vi "Verify Power Down.vi"(0 "Measurement Configuration":T3={"Quick Power Down"=FALSE, "Pin Name"=[], "Source Mode"=[], "Start Value"=[], "Target Value"=[], "Compliance Limit"=[], "Sense Mode"=[], "Default Ramp Rate"=[], "Ramp Rate"=[], "Start Delay"=[], "Relative To"=[], "Transient Response"=[], "Data Capture"=FALSE, "Power line frequency"=1} {"Relative To" items=["Power sequence start", "Previous source start", "Previous source end"]; "Power line frequency" items=["50 Hz", "60 Hz"]; "Start Value" format="%#_6p"; "Transient Response" items=["Slow", "Normal", "Fast"]; "Sense Mode" items=["Local Sense", "Remote Sense"]; "Target Value" format="%#_6p"; "Source Mode" items=["DC Voltage", "DC Current"]; "Start Delay" format="%#_6p"; "Compliance Limit" format="%#_6p"; "Ramp Rate" format="%#_6p"}, 5 "Measurements":T1, 7 "PowerUP?":bool, 11 "error in (no error)":errorcluster) -> (4 "Error[]":string[](array[string]), 15 "error out":errorcluster)   [LabVIEW 2024, in "devicePowerSequencerCoreLogic.lvlib"]
doc: "Checks status of pins to verify the power up"
uses:
  devicePowerSequencerCoreLogic.lvlib
  Measurement Configuration.ctl
  controls/Source Mode.ctl
  controls/Sense Mode.ctl
  controls/Relative To.ctl
  controls/Transient Response.ctl
  controls/Power line frequency.ctl
  controls/Measurements.ctl
  controls/Voltage and Current Measurements.ctl
  <vilib>/Utility/error.llb/Clear Errors.vi
  Form Error Message.vi/4da3fa3f-d6a2-4c6b-9c9c-fc44bca91f7b.vi
  <vilib>/Utility/error.llb/Error Cluster From Error Code.vi
  Device Power Sequencer.lvlib
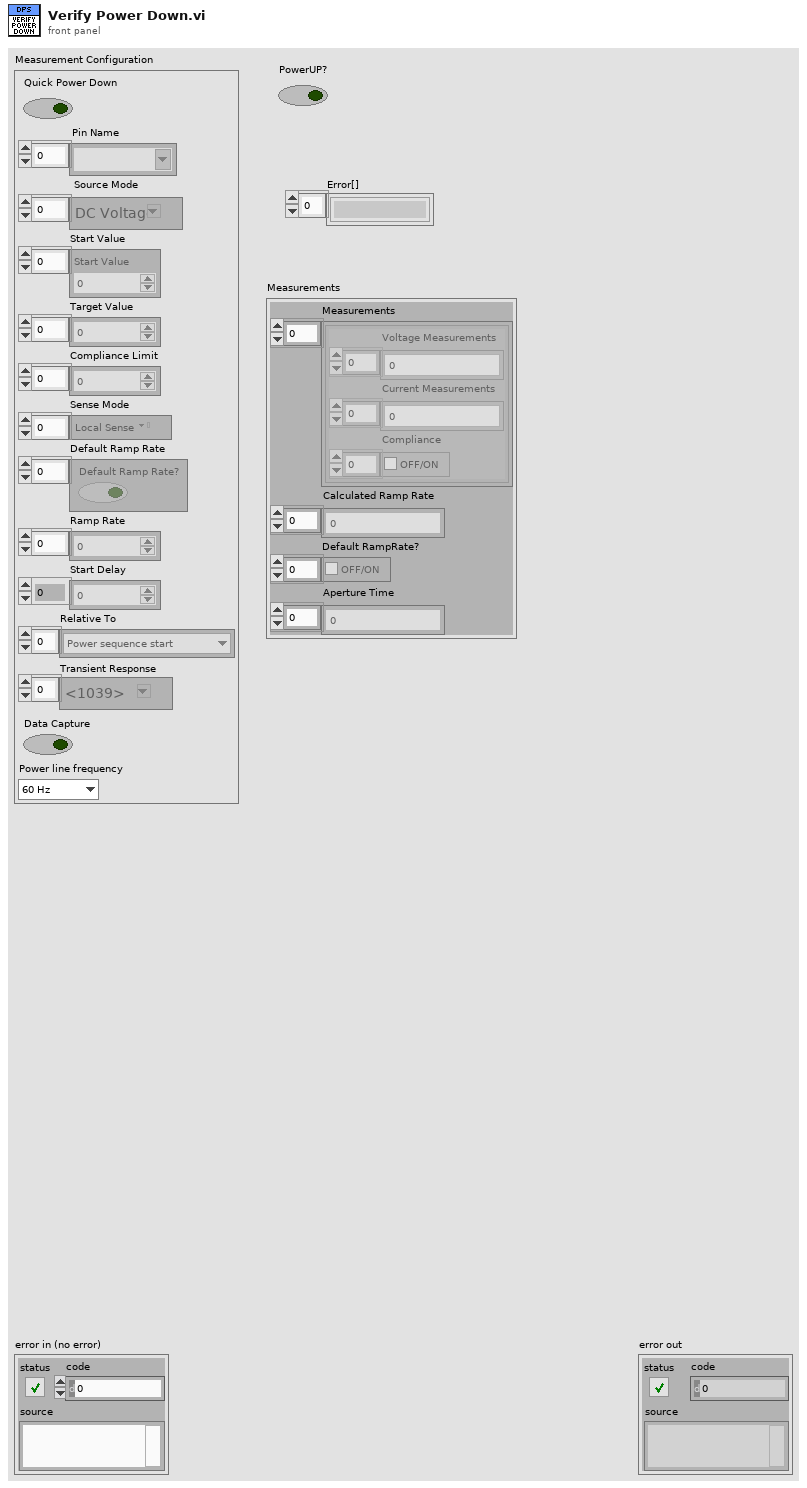
[diagram p1: front panel]
types:
  T1 = typedef "devicePowerSequencerCoreLogic.lvlib/Measurements.ctl" = cluster{"Measurements":T2[], "Calculated Ramp Rate":dbl[], "Default RampRate?":bool[], "Aperture Time":dbl[]}
  T2 = typedef "devicePowerSequencerCoreLogic.lvlib/Voltage and Current Measurements.ctl" = cluster{"Voltage Measurements":dbl[], "Current Measurements":dbl[], "Compliance":bool[]}
  T3 = typedef "Device Power Sequencer.lvlib/Measurement Configuration.ctl" = cluster{"Quick Power Down":bool, "Pin Name":string[], "Source Mode":T4[], "Start Value":dbl[], "Target Value":dbl[], "Compliance Limit":dbl[], "Sense Mode":T5[], "Default Ramp Rate":bool[], "Ramp Rate":dbl[], "Start Delay":dbl[], "Relative To":T6[], "Transient Response":T7[], "Data Capture":bool, "Power line frequency":T8}
  T4 = typedef "Device Power Sequencer.lvlib/Source Mode.ctl" = i32
  T5 = typedef "Device Power Sequencer.lvlib/Sense Mode.ctl" = i32
  T6 = typedef "Device Power Sequencer.lvlib/Relative To.ctl" = u32
  T7 = typedef "Device Power Sequencer.lvlib/Transient Response.ctl" = i32
  T8 = typedef "Device Power Sequencer.lvlib/Power line frequency.ctl" = u32
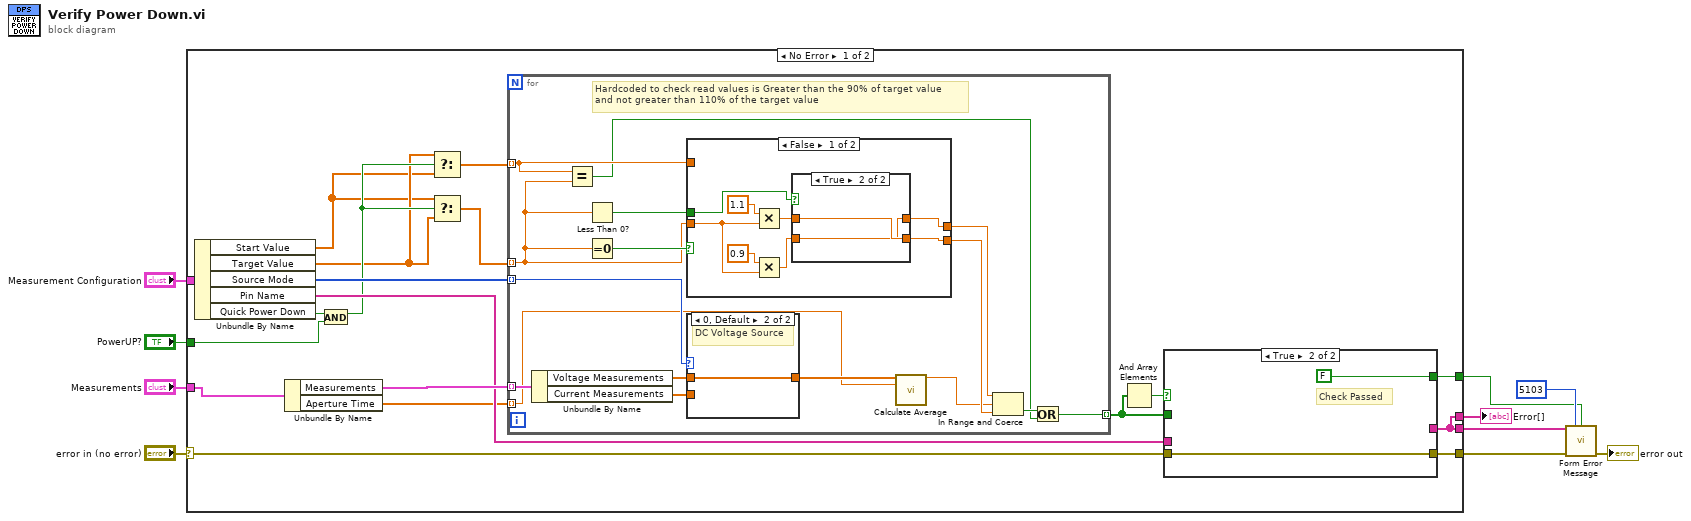
[diagram p0: block diagram]
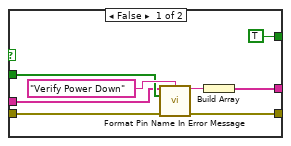
[diagram p2: hidden frame]
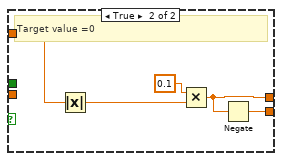
[diagram p4: hidden frame]
diagram:
  n1 = case shown="No Error" "error in (no error)" {
    selector: "error in (no error)" -> [w25 w75]
    tunnel: [w24 w75] -> w6
    tunnel: "Measurement Configuration" -> [w29 _]
    tunnel: "Measurements" -> [w27 _]
    tunnel: [w19 _] -> w4
    tunnel: [w20 _] -> w3
    tunnel: [w19 _] -> w2
    tunnel: "PowerUP?" -> [w14 _]
    frame No Error {
      n2 = Unbundle By Name(w29) -> ("Start Value"=w12:dbl[], "Target Value"=w13:dbl[], "Source Mode"=w28:T4[], "Pin Name"=w21:string[], "Quick Power Down"=w15:bool)
      n3 = Unbundle By Name(w27) -> ("Measurements"=w26:T2[], "Aperture Time"=w11:dbl[])
      n4 = And(x=w15, y=w14) -> (x .and. y?=w16:bool)
      n5 = Select(t=w13, s=w16, f=w12) -> (s? t:f=w18:dbl[])
      n6 = Select(t=w12, s=w16, f=w13) -> (s? t:f=w17:dbl[])
      n7 = for {
        tunnel: w26 -> [w55] mode=indexing
        tunnel: w28 -> [w54] mode=indexing
        tunnel: w17 -> [w44] mode=indexing
        tunnel: w18 -> [w45] mode=indexing
        tunnel: [w46] -> w22 mode=indexing
        tunnel: w11 -> [w41] mode=indexing
        # "Hardcoded to check read values is Greater than the 90% of target value\nand not greater than 110% of the target value"
        n8 = Unbundle By Name(w55) -> ("Voltage Measurements"=w52:dbl[], "Current Measurements"=w53:dbl[])
        n9 = Equal?(x=w45, y=w44) -> (x = y?=w43:bool)
        n10 = Less Than 0?(x=w44) -> (x < 0?=w48:bool)
        n11 = Equal To 0?(x=w44) -> (x = 0?=w49:bool)
        n12 = case shown="False" w49 {
          tunnel: [w59 w71] -> w51
          tunnel: [w58 w70] -> w50
          tunnel: w44 -> [w57 _]
          tunnel: w45 -> [_ w69]
          tunnel: w48 -> [w56 _]
          frame False {
            n13 = Multiply(x=1.1, y=w57) -> (x*y=w61:dbl)
            n14 = Multiply(x=0.9, y=w57) -> (x*y=w60:dbl)
            n15 = case shown="True" w56 {
              tunnel: w61 -> [w65 w67]
              tunnel: [w65 w66] -> w59
              tunnel: w60 -> [w64 w66]
              tunnel: [w64 w67] -> w58
              frame False {
              }
              frame True {
              }
            }
          }
          frame True {
            # "Target value =0"
            n16 = Absolute Value(x=w69) -> (abs(x)=w68:dbl)
            n17 = Multiply(x=0.1, y=w68) -> (x*y=w71:dbl)
            n18 = Negate(x=w71) -> (-x=w70:dbl)
          }
        }
        n19 = case shown="0, Default" w54 {
          tunnel: w53 -> [w73 _]
          tunnel: w52 -> [_ w74]
          tunnel: [w73 w74] -> w42
          frame 1 {
            # "DC Current Source"
          }
          frame 0, Default {
            # "DC Voltage Source"
          }
        }
        n20 = call "Calculate Average.vi"("Measurements"=w42, "Aperture Time"=w41) -> ("Average level"=w40:dbl)  [unwired: 13 in]
        n21 = In Range and Coerce(upper limit=w51, x=w40, lower limit=w50) -> (In Range?=w47:bool)  [unwired: 1 out]
        n22 = Or(x=w47, y=w43) -> (x .or. y?=w46:bool)
      }
      n23 = And Array Elements(Boolean array=w22) -> (logical AND=w23:bool)
      n24 = case shown="True" w23 {
        tunnel: [w36 w38] -> w24
        tunnel: [w35 _] -> w19
        tunnel: [TRUE ("Boolean") FALSE ("Boolean")] -> w20
        tunnel: w25 -> [w32 w38]
        tunnel: w22 -> [w31 _]
        tunnel: w21 -> [w30 _]
        frame False {
          n25 = call "Format Pin Name In Error Message.vi"("Pin Name"=w30, "Parameter Name"="Verify Power Down", "Error[]"=w31, "error in"=w32) -> ("Error Message"=w37:string, "error out"=w36:errorcluster)  [unwired: 10 in]
          n26 = Build Array(w37) -> (w35:string[])
        }
        frame True {
          # "Check Passed"
        }
      }
    }
    frame Error {
    }
  }
  "Error[]" <- w4
  n27 = call "Form Error Message.vi"("Error Message"=w2, "error code (0)"=5103, "Error?"=w3, "error in (no error)"=w6) -> ("error out"=→"error out":errorcluster)  [unwired: 11 in]
